vi "Create_Object.vi"(8 "error in (no error)":errorcluster, 9 "Block Diagram in":T1, 10 "owner refnum":variant, 11 "Array Constant in":refnum<class "Array Constant.lvclass">) -> (0 "error out":errorcluster, 1 "Block Diagram Out":T1, 3 "Array Constant out":refnum<class "Array Constant.lvclass">)   [LabVIEW 2025, in "Array Constant.lvclass"]
uses:
  Array Constant.lvclass
  C:/Users/mrjak/Documents/GitHub/LVGPT/LabVIEW/VIs/Classes/Node/Node.lvclass
  Controls/bd.ctl
  Node.lvclass
  Controls/wire.ctl
  Controls/Terminal.ctl
  Node.lvclass/Node.ctl
  Array.lvclass
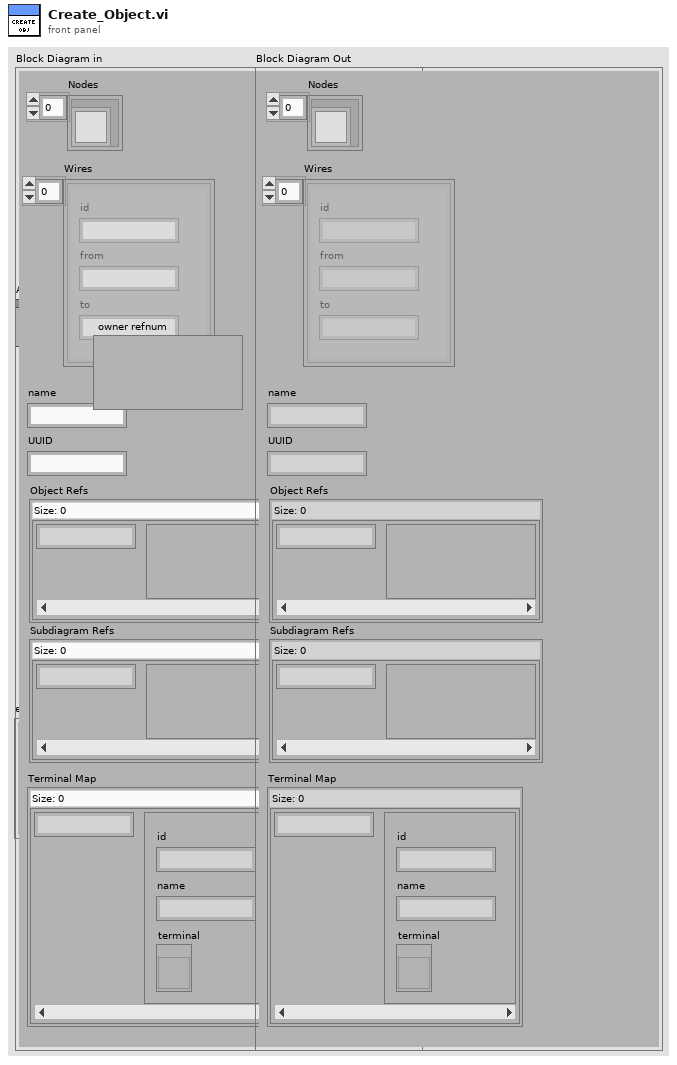
[diagram p1: front panel]
types:
  T1 = typedef "bd.ctl" = cluster{"Nodes":refnum<class "Node.lvclass">[], "Wires":T2[], "name":string, "UUID":string, "Object Refs":map{string, variant}, "Subdiagram Refs":map{string, variant}, "Terminal Map":map{string, T3}}
  T2 = typedef "wire.ctl" = cluster{"id":string, "from":string, "to":string}
  T3 = typedef "Terminal.ctl" = cluster{"id":string, "name":string, "terminal":refnum<vi>}
  T4 = typedef "LVPointTypeDef.ctl" = cluster{"Horizontal":i16, "Vertical":i16}
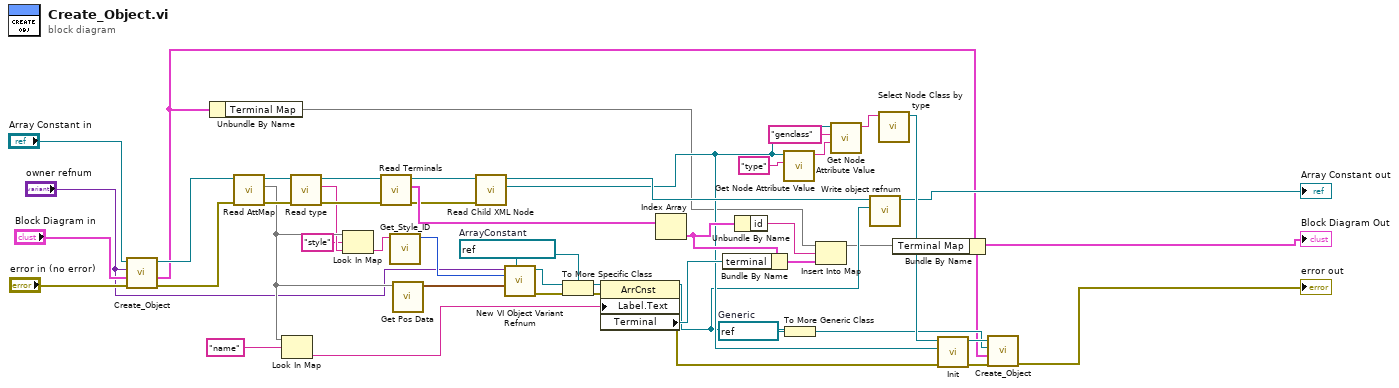
[diagram p0: block diagram]
diagram:
  w14 = refnum<vi> refnum  # Generic
  w11 = refnum<vi> refnum  # ArrayConstant
  n1 = call-parent "Create_Object.vi"("error in (no error)"="error in (no error)", "Block Diagram in"="Block Diagram in", "owner refnum"="owner refnum", "Node in"="Array Constant in") -> ("error out"=w7:errorcluster, "Block Diagram Out"=w3:T1, "Node out"=w8:refnum<class "Array Constant.lvclass">)  [unwired: 5 in]
  n2 = Unbundle By Name(w3) -> ("Terminal Map"=w4:map{string, T3})
  n3 = call "Read AttMap.vi"("error in (no error)"=w7, "Node in"=w8) -> ("error out"=w44:errorcluster, "AttMap"=w24:map{string, string}, "Node out"=w43:refnum<class "Array Constant.lvclass">)  [unwired: 7 in]
  n4 = Look In Map(map=w24, key="name") -> (value=w36:string)  [unwired: 1 in, 1 out]
  n5 = call "Read type.vi"("error in (no error)"=w44, "Node in"=w43) -> ("error out"=w41:errorcluster, "type"=w23:string, "Node out"=w40:refnum<class "Array Constant.lvclass">)  [unwired: 7 in]
  n6 = Look In Map(map=w24, key="style", default value=w23) -> (value=w21:string)  [unwired: 1 out]
  n7 = call "Read Terminals.vi"("error in (no error)"=w41, "Node in"=w40) -> ("error out"=w30:errorcluster, "Terminals"=w31:T3[], "Node out"=w29:refnum<class "Array Constant.lvclass">)  [unwired: 7 in]
  n8 = call "Get_Style_ID.vi"("Style"=w21) -> ("style"=w42:i32)  [unwired: 8 in, 2 out]
  n9 = call "Get Pos Data.vi"("AttMap"=w24) -> ("Position"=w45:T4)  [unwired: 10 in]
  n10 = call-dynamic "Read Child XML Node.vi"("error in (no error)"=w30, "Array in"=w29) -> ("Child XML Node"=w17:refnum<k20>, "Array out"=w25:refnum<class "Array Constant.lvclass">)  [unwired: 7 in, 1 out]
  n11 = call "New VI Object Variant Refnum.vi"("vi object class"=w11, "location"=w45, "style"=w42, "owner refnum"="owner refnum") -> ("error out"=w37:errorcluster, "object refnum"=w38:refnum<vi>)  [unwired: 6 in]
  n12 = To More Specific Class(target class=w11, reference=w38) -> (specific class reference=w12:refnum<vi>)  [unwired: 1 in, 1 out]
  n13 = property class="ArrCnst"(reference=w12, error in=w37, "Label.Text"=w36) -> (reference out=w10:refnum<vi>, error out=w18:errorcluster, "Terminal"=w32:refnum<vi>)
  n14 = Index Array(array=w31) -> (element=w34:T3)  [unwired: 1 in]
  n15 = Bundle By Name(cluster=w34, "terminal"=w32) -> (w33:T3)
  n16 = Unbundle By Name(w34) -> ("id"=w35:string)
  n17 = call "Get Node Attribute Value.vi"("Attribute Name"="type", "Refnum in"=w17) -> ("Value"=w27:string)  [unwired: 9 in]
  n18 = To More Generic Class(target class=w14, reference=w10) -> (generic class reference=w13:refnum<vi>)
  n19 = Insert Into Map(map in=w4, key=w35, value=w33) -> (map out=w2:map{string, T3})  [unwired: 2 out]
  n20 = call "Get Node Attribute Value.vi"("Default Value"=w27, "Attribute Name"="genclass", "Refnum in"=w17) -> ("Value"=w20:string)  [unwired: 8 in]
  n21 = call-dynamic "Write object refnum.vi"("object refnum"=w10, "Node in"=w25) -> ("Node out"=→"Array Constant out":refnum<class "Array Constant.lvclass">)  [unwired: 8 in, 1 out]
  n22 = call "Select Node Class by type.vi"("Value"=w20) -> ("Node out"=w19:refnum<class "Node.lvclass">)  [unwired: 10 in]
  n23 = Bundle By Name(cluster=w3, "Terminal Map"=w2) -> (w1:T1)
  "Block Diagram Out" <- w1
  n24 = call-dynamic "Init.vi"("error in (no error)"=w18, "Node Reg"=w17, "Node in"=w19) -> ("error out"=w16:errorcluster, "Node out"=w15:refnum<class "Node.lvclass">)  [unwired: 7 in]
  n25 = call-dynamic "Create_Object.vi"("error in (no error)"=w16, "Block Diagram in"=w1, "owner refnum"=w13, "Node in"=w15) -> ("error out"=→"error out":errorcluster)  [unwired: 5 in, 2 out]
